vi "Write System Name.vi"(8 "error in":errorcluster, 10 "system name":string, 11 "cRIO in":refnum<class "cRIO.lvclass">) -> (0 "error out":errorcluster, 3 "cRIO out":refnum<class "cRIO.lvclass">)   [LabVIEW 2015, in "cRIO.lvclass"]
uses:
  cRIO.lvclass
  cRIO.lvclass/cRIO.ctl
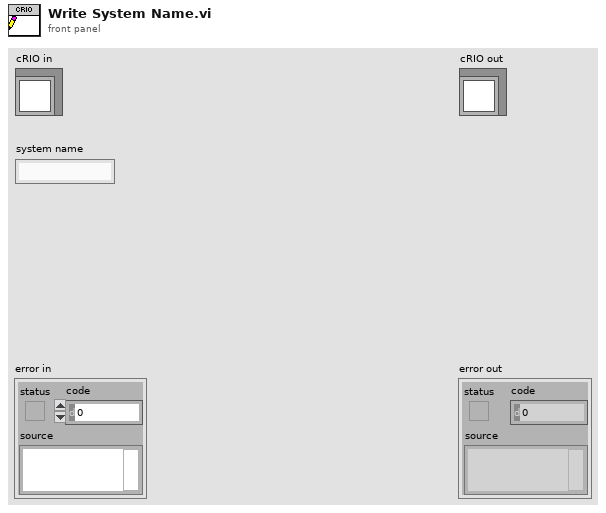
[diagram p1: front panel]
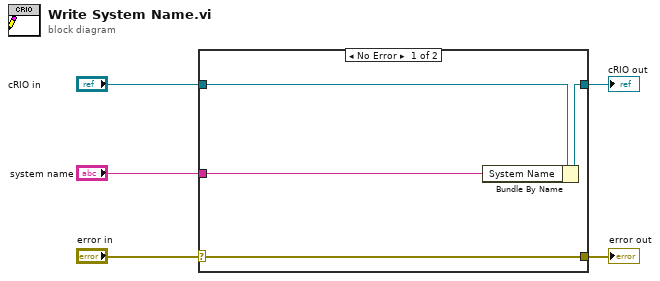
[diagram p0: block diagram]
diagram:
  n1 = case shown="No Error" "error in" {
    selector: "error in" -> [w9 w10]
    tunnel: [w9 w10] -> w4
    tunnel: [w7 w11] -> w2
    tunnel: "cRIO in" -> [w8 w11]
    tunnel: "system name" -> [w6 _]
    frame No Error {
      n2 = Bundle By Name(cluster=w8, "System Name"=w6) -> (w7:refnum<class "cRIO.lvclass">)
    }
    frame Error {
    }
  }
  "error out" <- w4
  "cRIO out" <- w2
